vi "마이크 스피커 출력 실습.vi"() -> ()   [LabVIEW 2020]
uses:
  <vilib>/DAQmx/read.llb/DAQmx Read (Analog Wfm 1Chan NSamp).vi
  <vilib>/DAQmx/write.llb/DAQmx Write (Analog Wfm 1Chan NSamp).vi
  <vilib>/DAQmx/create/channels.llb/DAQmx Create Channel (AI-Voltage-Basic).vi
  <vilib>/DAQmx/configure/timing.llb/DAQmx Timing (Sample Clock).vi
  <vilib>/DAQmx/miscellaneous.llb/DAQmx Fill In Error Info.vi
  <vilib>/DAQmx/create/channels.llb/DAQmx Create Channel (AO-Voltage-Basic).vi
  <vilib>/DAQmx/configure/timing.llb/DAQmx Timing (Use Waveform).vi
panel:
  out "숫자형":i32
  out "녹음 그래프":waveform(dbl)(graph)
  in  "정지":bool
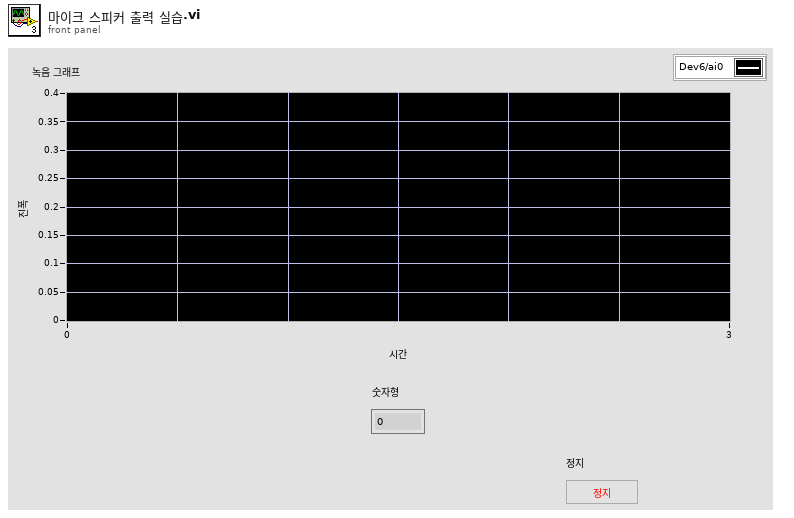
[diagram p1: front panel]
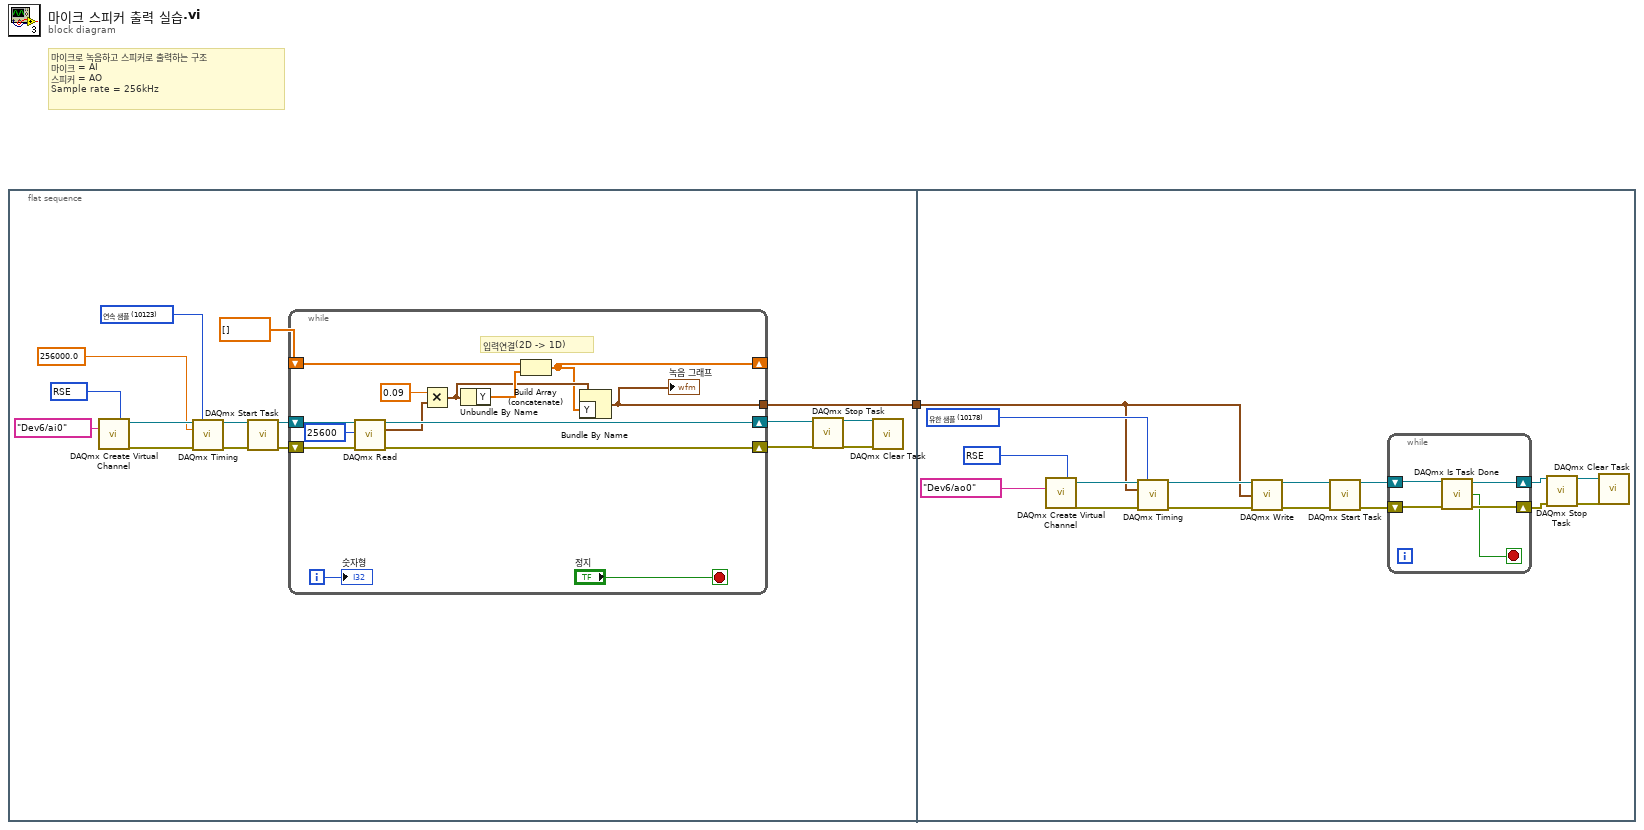
[diagram p0: block diagram]
diagram:
  # "마이크로 녹음하고 스피커로 출력하는 구조\n마이크 = AI\n스피커 = AO\nSample rate = 256kHz"
  n1 = flat-sequence {
    tunnel: [w7] -> w1
    tunnel: w1 -> [w39]
    frame #0 {
      w13 = 10123 items=["유한 샘플"=10178, "연속 샘플"=10123, "하드웨어 타이밍에 의한 단일 포인트"=12522] ("sample mode")
      w16 = 10083 items=["기본"=-1, "RSE"=10083, "NRSE"=10078, "차동"=10106, "유사 차동"=12529] ("input terminal configuration")
      n2 = call-poly <vilib>:"DAQmx Create Virtual Channel.vi"("input terminal configuration"=w16, "physical channels"=tag "Dev6/ai0") -> ("task out"=w15:refnum<k21>, "error out"=w14:errorcluster)  [unwired: 12 in]
      n3 = call-poly <vilib>:"DAQmx Timing.vi"("task/channels in"=w15, "sample mode"=w13, "rate"=256000.0, "error in"=w14) -> ("task out"=w12:refnum<k21>, "error out"=w11:errorcluster)  [unwired: 10 in]
      n4 = call <vilib>:"DAQmx Start Task.vi"("task/channels in"=w12, "error in"=w11) -> ("task out"=w10:refnum<k21>, "error out"=w9:errorcluster)  [unwired: 12 in]
      n5 = while {
        shift-right: [w29] -> w6
        shift-left: w10 -> [w31]
        shift-right: [w28] -> w5
        shift-left: w9 -> [w30]
        shift-right: [w21] -> _
        shift-left: dbl[] [] -> [w24]
        tunnel: [w20] -> w7
        i -> [w18]
        stop <- "정지" stop-if-true
        # "입력연결(2D -> 1D)"
        n6 = call-poly <vilib>:"DAQmx Read.vi"("task/channels in"=w31, "number of samples per channel"=25600, "error in"=w30) -> ("task out"=w29:refnum<k21>, "data"=w26:waveform(dbl), "error out"=w28:errorcluster)  [unwired: 10 in]
        n7 = Multiply(x=0.09, y=w26) -> (x*y=w22:waveform(dbl))
        n8 = Unbundle By Name(w22) -> ("Y"=w23:dbl[])
        n9 = Build Array (concatenate)(w24, w23) -> (w21:dbl[])
        n10 = Bundle By Name(cluster=w22, "Y"=w21) -> (w20:waveform(dbl))
        "녹음 그래프" <- w20
        "숫자형" <- w18
      }
      n11 = call <vilib>:"DAQmx Stop Task.vi"("task/channels in"=w6, "error in"=w5) -> ("task out"=w4:refnum<k21>, "error out"=w3:errorcluster)  [unwired: 12 in]
      n12 = call <vilib>:"DAQmx Clear Task.vi"("task in"=w4, "error in"=w3) -> ()  [unwired: 13 in, 1 out]
    }
    frame #1 {
      w44 = 10178 items=["유한 샘플"=10178, "연속 샘플"=10123, "하드웨어 타이밍에 의한 단일 포인트"=12522] ("sample mode")
      w45 = 10083 items=["기본"=-1, "RSE"=10083, "NRSE"=10078, "차동"=10106, "유사 차동"=12529] ("input terminal configuration")
      n13 = call-poly <vilib>:"DAQmx Create Virtual Channel.vi"("output terminal configuration"=w45, "physical channels"=tag "Dev6/ao0") -> ("task out"=w43:refnum<k21>, "error out"=w42:errorcluster)  [unwired: 12 in]
      n14 = call-poly <vilib>:"DAQmx Timing.vi"("task/channels in"=w43, "sample mode"=w44, "waveform"=w39, "error in"=w42) -> ("task out"=w41:refnum<k21>, "error out"=w40:errorcluster)  [unwired: 10 in]
      n15 = call-poly <vilib>:"DAQmx Write.vi"("task/channels in"=w41, "data"=w39, "error in"=w40) -> ("task out"=w38:refnum<k21>, "error out"=w37:errorcluster)  [unwired: 10 in, 1 out]
      n16 = call <vilib>:"DAQmx Start Task.vi"("task/channels in"=w38, "error in"=w37) -> ("task out"=w36:refnum<k21>, "error out"=w35:errorcluster)  [unwired: 12 in]
      n17 = while {
        shift-right: [w49] -> w34
        shift-left: w36 -> [w52]
        shift-right: [w50] -> w33
        shift-left: w35 -> [w51]
        stop <- w48 stop-if-true
        n18 = call <vilib>:"DAQmx Is Task Done.vi"("task/channels in"=w52, "error in"=w51) -> ("task out"=w49:refnum<k21>, "task done?"=w48:bool, "error out"=w50:errorcluster)  [unwired: 11 in]
      }
      n19 = call <vilib>:"DAQmx Stop Task.vi"("task/channels in"=w34, "error in"=w33) -> ("task out"=w47:refnum<k21>, "error out"=w46:errorcluster)  [unwired: 12 in]
      n20 = call <vilib>:"DAQmx Clear Task.vi"("task in"=w47, "error in"=w46) -> ()  [unwired: 13 in, 1 out]
    }
  }
